vi "Write to File.vi"(8 "error in (no error)":errorcluster, 9 "Max File Size (bytes)":i64, 10 "Log Message":string, 11 "Error Log":path) -> (0 "error out":errorcluster)   [LabVIEW 2019, in "TSC Error.lvlib" / "ERROR_Write.lvclass"]
doc: "Write the error text file information while checking if the file is bigger than the maximum size.\n\n<b>Code Developed By:</b>\nCyril Rybicki\nTechnology Service Corporation\n1983 S Liberty Drive\nBloomington, IN 47403\nwww.tsc.com/atcs"
uses:
  ERROR_Write.lvclass
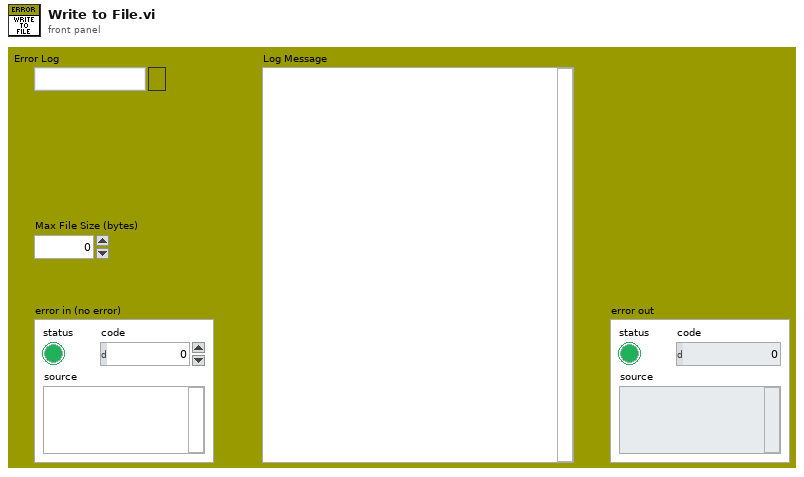
[diagram p1: front panel]
types:
  T1 = enum16{"open", "replace", "create", "open or create", "replace or create", "replace or create with confirmation"}
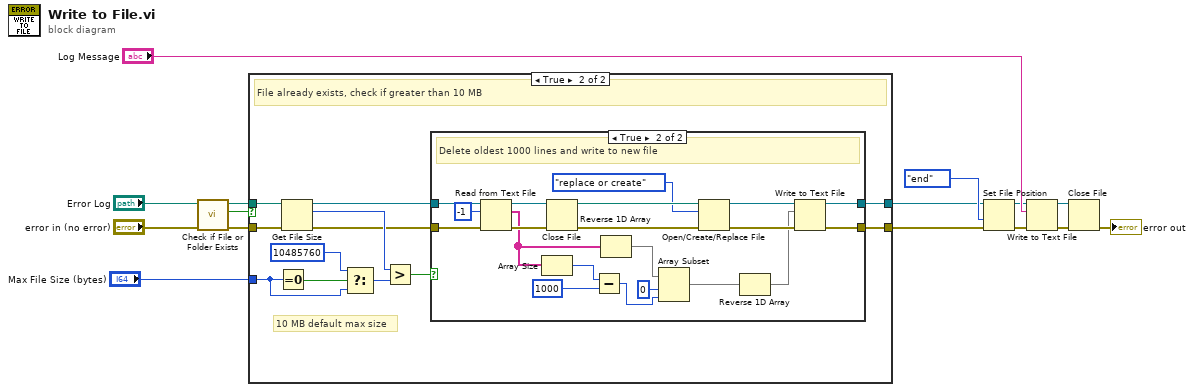
[diagram p0: block diagram]
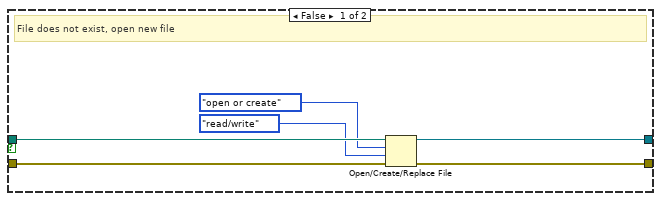
[diagram p2: hidden frame]
diagram:
  n1 = call <vilib>:"Check if File or Folder Exists.vi"("error in (no error)"="error in (no error)", "path"="Error Log") -> ("error out"=w7:errorcluster, "file or folder exists?"=w4:bool, "dup path"=w5:path)  [unwired: 7 in]
  n2 = case shown="True" w4 {
    tunnel: w7 -> [w20 w30]
    tunnel: w5 -> [w21 w29]
    tunnel: [w19 w27] -> w3
    tunnel: [w18 w26] -> w2
    tunnel: "Max File Size (bytes)" -> [_ w23]
    frame False {
      # "File does not exist, open new file"
      n3 = Open/Create/Replace File(file path (use dialog)=w21, error in=w20, operation (0:open)=T1."open or create", access (0:read/write)=enum16{"read/write", "read-only", "write-only"}."read/write") -> (refnum out=w19:refnum<file>, error out=w18:errorcluster)  [unwired: 2 in, 1 out]
    }
    frame True {
      # "10 MB default max size"
      # "File already exists, check if greater than 10 MB"
      n4 = Equal To 0?(x=w23) -> (x = 0?=w24:bool)
      n5 = Get File Size(file=w29, error in=w30) -> (refnum out=w31:refnum<file>, size (in bytes)=w33:i64, 0:w28:errorcluster)
      n6 = Select(t=i64 10485760 ("y"), s=w24, f=w23) -> (s? t:f=w22:i64)
      n7 = Greater?(x=w33, y=w22) -> (0:w32:bool)
      n8 = case shown="True" w32 {
        tunnel: w31 -> [w35 w55]
        tunnel: w28 -> [w34 w54]
        tunnel: [w35 w37] -> w27
        tunnel: [w34 w36] -> w26
        frame False {
          # "Less than 10 MB, no action needed"
        }
        frame True {
          # "Delete oldest 1000 lines and write to new file"
          n9 = Read from Text File(file (use dialog)=w55, count=-1, error in=w54) -> (refnum out=w47:refnum<file>, text=w45:string[], error out=w46:errorcluster)  [unwired: 1 in, 1 out]
          n10 = Array Size(array=w45) -> (size(s)=w50:i32)
          n11 = Close File(refnum=w47, error in=w46) -> (path=w43:path, error out=w42:errorcluster)
          n12 = Subtract(x=w50, y=1000 ("length")) -> (x-y=w52:i32)
          n13 = Reverse 1D Array(array=w45) -> (reversed array=w44:string[])
          n14 = Array Subset "Array Subset"(array=w44, index=0, length=w52) -> (w48:string[])
          n15 = Open/Create/Replace File(file path (use dialog)=w43, error in=w42, operation (0:open)=T1."replace or create") -> (refnum out=w40:refnum<file>, error out=w39:errorcluster)  [unwired: 3 in, 1 out]
          n16 = Reverse 1D Array(array=w48) -> (reversed array=w38:string[])
          n17 = Write to Text File(file (use dialog)=w40, text=w38, error in=w39) -> (refnum out=w37:refnum<file>, error out=w36:errorcluster)  [unwired: 1 in, 1 out]
        }
      }
    }
  }
  n18 = Set File Position(refnum=w3, from (0:start)=enum16{"start", "end", "current"}."end", error in=w2) -> (refnum out=w8:refnum<file>, error out=w10:errorcluster)  [unwired: 1 in]
  n19 = Write to Text File(file (use dialog)=w8, text="Log Message", error in=w10) -> (refnum out=w12:refnum<file>, error out=w11:errorcluster)  [unwired: 1 in, 1 out]
  n20 = Close File(refnum=w12, error in=w11) -> (error out=→"error out":errorcluster)  [unwired: 1 out]
